vi "getBSONElement.vi"(7 "Name":string, 8 "error in (no error)":errorcluster, 11 "tBSONDocument in":refnum<class "tBSONDocument.lvclass">) -> (0 "error out":errorcluster, 2 "Element":refnum<class "tBSONElement.lvclass">, 3 "tBSONDocument out":refnum<class "tBSONDocument.lvclass">)   [LabVIEW 2013, in "BSON.lvlib" / "tBSONDocument.lvclass"]
doc: "Retrieves a BSON element from a BSON document."
uses:
  tBSONDocument.lvclass
  tBSONElement/tBSONElement.lvclass
  tBSONDocument.lvclass/tBSONDocument.ctl
  status.ctl
  BSONElements/tBSONDocumentElement/tBSONDocumentElement.lvclass
  BSONElements/tBSONDocumentElement/getValue.vi
  BSON.lvlib
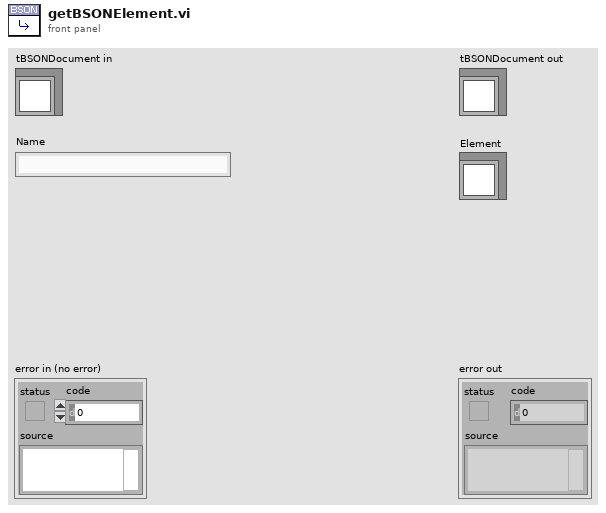
[diagram p1: front panel]
types:
  T1 = typedef "BSON.lvlib/status.ctl" = enum16{"Stream Corrupted or Ended Abruptly", "Incorrect Type In Stream", "ObjectID Invalid", "Method Not Implemented", "Invalid Name", "Invalid URI", "AutoReconnect", "Operation Failed", "Incorrectly Configured", "Cursor Not Found", "Timeout", "Invalid Type", "Empty Name", "Duplicate Name", "MD5Incorrect"}
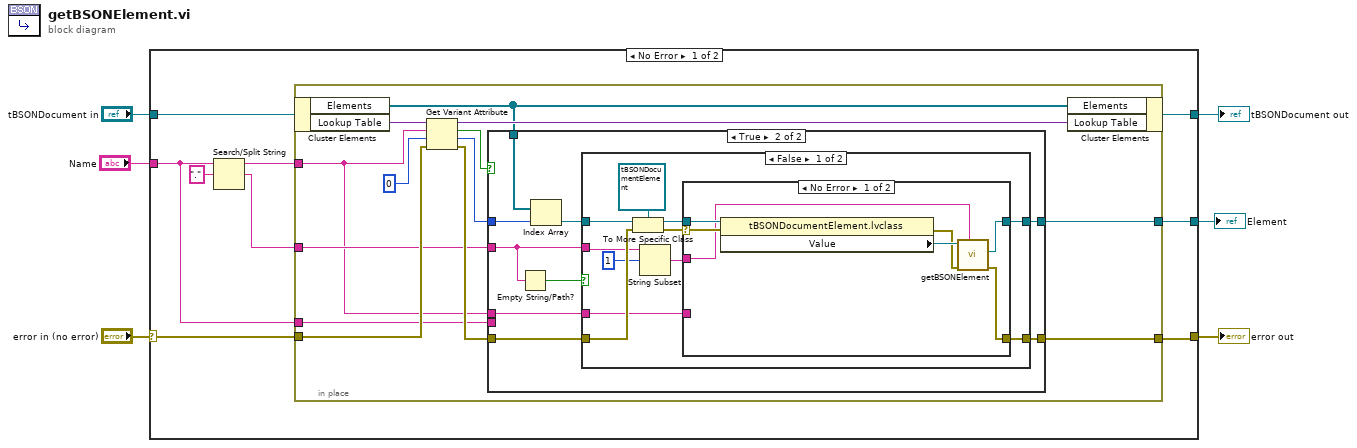
[diagram p0: block diagram]
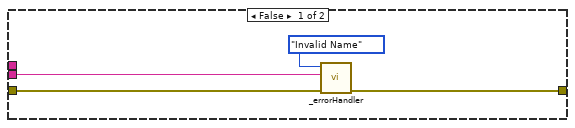
[diagram p2: hidden frame]
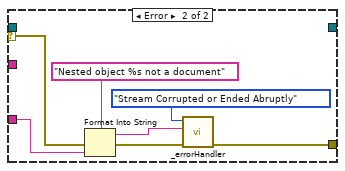
[diagram p3: hidden frame]
diagram:
  n1 = case shown="No Error" "error in (no error)" {
    selector: "error in (no error)" -> [w14 w70]
    tunnel: [w9 w70] -> w5
    tunnel: [w7 w69] -> w3
    tunnel: "tBSONDocument in" -> [w12 w69]
    tunnel: "Name" -> [w8 _]
    tunnel: [w10 _] -> w1
    frame No Error {
      n2 = Search/Split String(string=w8, search string/char (-)=".") -> (substring before match=w13:string, match + rest of string=w11:string)  [unwired: 1 in, 1 out]
      n3 = in-place {
        in-place-border: w14 -> [w27]
        in-place-border: w13 -> [w16]
        in-place-border: w11 -> [w21]
        in-place-border: [w20] -> w10
        in-place-border: [w19] -> w9
        in-place-border: w8 -> [w17]
        n4 = in-place-cluster #1(w12) -> ("Elements"=w18:refnum<class "tBSONElement.lvclass">[], "Lookup Table"=w28:variant)
        n5 = Get Variant Attribute(Variant=w28, name=w16, default value (empty Variant)=0, error in=w27) -> (duplicate Variant=w25:variant, found=w24:bool, value=w22:i32, error out=w23:errorcluster)
        n6 = case shown="True" w24 {
          tunnel: w23 -> [w32 w39]
          tunnel: w22 -> [_ w41]
          tunnel: w21 -> [_ w34]
          tunnel: [_ w37] -> w20
          tunnel: [w29 w36] -> w19
          tunnel: w18 -> [_ w35]
          tunnel: w17 -> [w30 _]
          tunnel: w16 -> [_ w33]
          frame False {
            n7 = call "_errorHandler.vi"("error in (no error)"=w32, "Additional Text"=w30, "Error Type"=status."Invalid Name") -> ("error out"=w29:errorcluster)  [unwired: 8 in]
          }
          frame True {
            n8 = Empty String/Path?(string/path=w34) -> (empty?=w40:bool)
            n9 = Index Array(array=w35, index=w41) -> (element=w38:refnum<class "tBSONElement.lvclass">)
            n10 = case shown="False" w40 {
              tunnel: w39 -> [w50 w67]
              tunnel: w38 -> [w52 w68]
              tunnel: [w46 w68] -> w37
              tunnel: [w47 w67] -> w36
              tunnel: w34 -> [w44 _]
              tunnel: w33 -> [w45 _]
              frame False {
                n11 = To More Specific Class(target class=refnum<class "tBSONDocumentElement.lvclass"> refnum ("BSON.lvlib:tBSONDocumentElement.lvclass"), reference=w52, error in=w50) -> (specific class reference=w48:refnum<class "tBSONDocumentElement.lvclass">, error out=w49:errorcluster)
                n12 = String Subset(string=w44, offset (0)=1) -> (substring=w42:string)  [unwired: 1 in]
                n13 = case shown="No Error" w49 {
                  selector: w49 -> [w59 w64]
                  tunnel: w48 -> [w58 _]
                  tunnel: w42 -> [w53 _]
                  tunnel: [w55 w65] -> w47
                  tunnel: [w54 _] -> w46
                  tunnel: w45 -> [_ w62]
                  frame No Error {
                    n14 = property class="tBSONDocumentElement.lvclass"(reference=w58, error in=w59) -> (error out=w56:errorcluster, "Value"=w57:refnum<class "tBSONDocument.lvclass">)  [unwired: 1 out]
                    n15 = call "getBSONElement.vi"("Name"=w53, "error in (no error)"=w56, "tBSONDocument in"=w57) -> ("error out"=w55:errorcluster, "Element"=w54:refnum<class "tBSONElement.lvclass">)  [unwired: 6 in, 1 out]
                  }
                  frame Error {
                    n16 = Format Into String(format string="Nested object %s not a document" ("Additional Text"), error in=w64, w62) -> (resulting string=w61:string, error out=w60:errorcluster)  [unwired: 1 in]
                    n17 = call "_errorHandler.vi"("error in (no error)"=w60, "Additional Text"=w61, "Error Type"=status."Stream Corrupted or Ended Abruptly") -> ("error out"=w65:errorcluster)  [unwired: 8 in]
                  }
                }
              }
              frame True {
              }
            }
          }
        }
        n18 = in-place-cluster #1("Elements"=w18, "Lookup Table"=w25) -> (w7:refnum<class "tBSONDocument.lvclass">)
      }
    }
    frame Error {
    }
  }
  "error out" <- w5
  "tBSONDocument out" <- w3
  "Element" <- w1
